vi "test.vi"() -> ()   [LabVIEW 2011]
panel:
  out "error out":errorcluster
  out "path":path
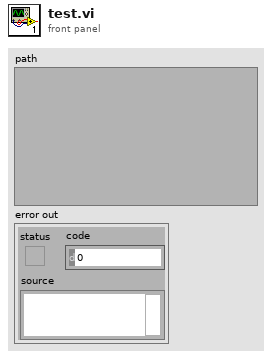
[diagram p1: front panel]
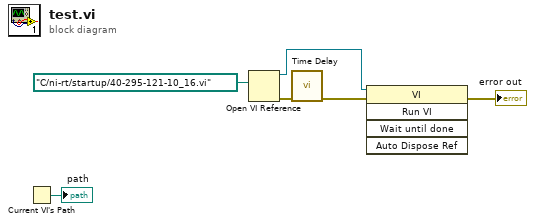
[diagram p0: block diagram]
diagram:
  n1 = Current VI's Path() -> (path=→"path":path)
  n2 = Open VI Reference(vi path=path "C:/ni-rt/startup/40-295-121-10_16.vi" ("path 2")) -> (vi reference=w3:refnum<vi>, error out=w2:errorcluster)  [unwired: 5 in]
  n3 = call "Time Delay"("error in (no error)"=w2) -> ("error out"=w1:errorcluster)  [unwired: 10 in]
  n4 = invoke class="VI" method="Run VI"(reference=w3, error in=w1) -> (error out=→"error out":errorcluster)  [unwired: 3 in, 4 out]
